vi "Ke2000 Initialize.vi"(8 "error in (no error)":errorcluster, 9 "Default Setting":bool, 10 "Reset":bool, 11 "VISA resource name":refnum<visa-resource-name>) -> (0 "error out":errorcluster, 3 "VISA resource name out":refnum<visa-resource-name>)   [LabVIEW 2017]
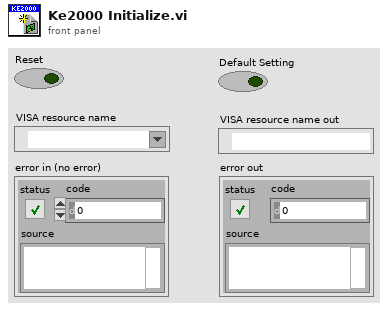
[diagram p1: front panel]
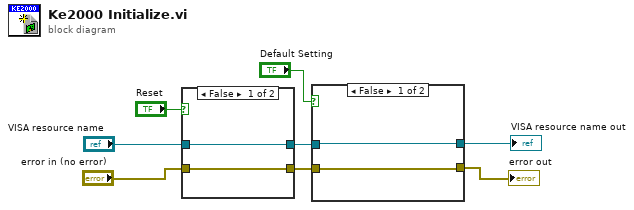
[diagram p0: block diagram]
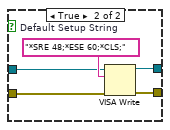
[diagram p2: hidden frame]
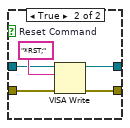
[diagram p3: hidden frame]
diagram:
  n1 = case shown="False" "Reset" {
    tunnel: [w10 w14] -> w8
    tunnel: "VISA resource name" -> [w10 w13]
    tunnel: "error in (no error)" -> [w9 w12]
    tunnel: [w9 w11] -> w5
    frame False {
    }
    frame True {
      w15 = "*RST;"  # Reset Command
      n2 = VISA Write(VISA resource name=w13, write buffer=w15, error in (no error)=w12) -> (VISA resource name out=w14:refnum<visa-resource-name>, error out=w11:errorcluster)  [unwired: 1 out]
    }
  }
  n3 = case shown="False" "Default Setting" {
    tunnel: w8 -> [w16 w21]
    tunnel: w5 -> [w17 w20]
    tunnel: [w17 w19] -> w4
    tunnel: [w16 w18] -> w3
    frame False {
    }
    frame True {
      w22 = "*SRE 48;*ESE 60;*CLS;"  # Default Setup String
      n4 = VISA Write(VISA resource name=w21, write buffer=w22, error in (no error)=w20) -> (VISA resource name out=w18:refnum<visa-resource-name>, error out=w19:errorcluster)  [unwired: 1 out]
    }
  }
  "error out" <- w4
  "VISA resource name out" <- w3
